vi "SubPanelTypecast.vi"(0 "Ctl Refnum":refnum<vi>, 7 "Control Path In":string[](array[string]), 11 "Error In":errorcluster) -> (4 "Controls[]":refnum<vi>[](array[refnum]), 8 "Control Path Out":string[](array[string]), 15 "Error Out":errorcluster)   [LabVIEW 2016]
uses:
  main/Drona.lvlib
  main/apis/Setup/GetControlRef/GetControlRef.lvlib
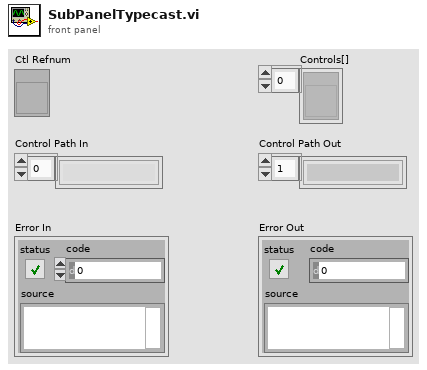
[diagram p1: front panel]
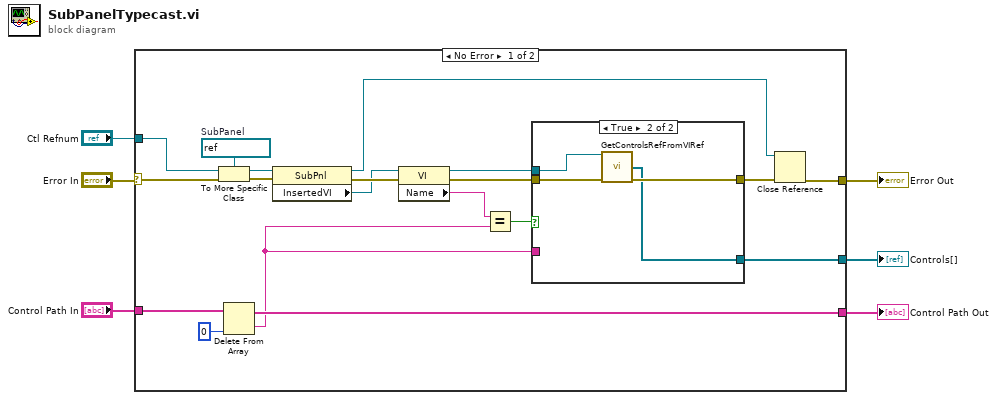
[diagram p0: block diagram]
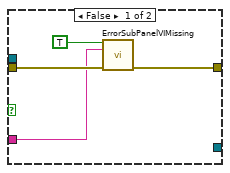
[diagram p2: hidden frame]
diagram:
  n1 = case shown="No Error" "Error In" {
    selector: "Error In" -> [w8 w35]
    tunnel: "Control Path In" -> [w25 w34]
    tunnel: "Ctl Refnum" -> [w7 _]
    tunnel: [w18 _] -> w4
    tunnel: [w17 w34] -> w3
    tunnel: [w16 w35] -> w2
    frame No Error {
      w22 = refnum<vi> refnum  # SubPanel
      n2 = To More Specific Class(target class=w22, reference=w7, error in=w8) -> (specific class reference=w24:refnum<vi>, error out=w23:errorcluster)
      n3 = Delete From Array(array=w25, index=0) -> (deleted portion=w10:string, array with subset deleted=w17:string[])  [unwired: 1 in]
      n4 = property class="SubPnl"(reference=w24, error in=w23) -> (reference out=w20:refnum<vi>, error out=w21:errorcluster, "InsertedVI"=w9:refnum<vi>)
      n5 = property class="VI"(reference=w9, error in=w21) -> (reference out=w12:refnum<vi>, error out=w13:errorcluster, "Name"=w15:string)
      n6 = Equal?(x=w15, y=w10) -> (x = y?=w14:bool)
      n7 = case shown="True" w14 {
        tunnel: w13 -> [w29 w32]
        tunnel: [w28 w31] -> w11
        tunnel: w12 -> [_ w33]
        tunnel: [_ w30] -> w18
        tunnel: w10 -> [w27 _]
        frame False {
          n8 = call "ErrorSubPanelVIMissing.vi"("Create Error?"=TRUE, "VI Name"=w27, "error in"=w29) -> ("error out"=w28:errorcluster)  [unwired: 12 in]
        }
        frame True {
          n9 = call "GetControlsRefFromVIRef.vi"("VI Reference In"=w33, "Error In"=w32) -> ("Controls[]"=w30:refnum<vi>[], "Error Out"=w31:errorcluster)  [unwired: 11 in, 1 out]
        }
      }
      n10 = Close Reference(reference=w20, error in (no error)=w11) -> (error out=w16:errorcluster)
    }
    frame Error {
    }
  }
  "Controls[]" <- w4
  "Control Path Out" <- w3
  "Error Out" <- w2
